vi "UHR-Fleezers Control (host) - 12.2.vi"() -> ()   [LabVIEW 2012] (continued)
      tunnel: [w2214] -> w1523 mode=indexing
      tunnel: w1485 -> [w2213]
      workers-P: _ -> [_]
      n1078 = Bundle By Name("Y"=w2218, "dt"=w2217) -> (w2219:waveform(dbl))  [unwired: 1 out]
      n1079 = Set Waveform Attribute(5:w2216, 6:w2215, 7:w2219) -> (3:w2214:waveform(dbl))  [unwired: 1 in, 2 out]
      n1080 = call "downsample 1D array - double.vi"("Ave N"=w2220, "Array In"=w2218) -> ("Array Out"=w2221:dbl[])  [unwired: 1 out]
      n1081 = Bundle By Name(cluster=w2214, "t0"=w2212, "Y"=w2221, "dt"=w2213) -> (w2222:waveform(dbl))
    }
    n1082 = Bundle("BD 1 Frequency 1 (MHz)"=w1439, "BD 1 Frequency 2 (MHz)"=w1438) -> (w1440:T41)  [unwired: 1 out]
    n1083 = call-poly <vilib>:"Mean.vi"("X"=w1473) -> ("mean"=w1461:dbl)  [unwired: 1 out]
    n1084 = call-poly <vilib>:"Mean.vi"("X"=w1474) -> ("mean"=w1462:dbl)  [unwired: 1 out]
    n1085 = Reciprocal(x=w1485) -> (1/x=→"Trap Disp. Freq. (Hz)":dbl)
    n1086 = Cluster To Array(cluster=w1440) -> (array=w1437:dbl[])
    n1087 = local read "Trap X AI1 (DMA)"() -> (w1472:T13)
    n1088 = local read "Data points/scans (MCL)"() -> (w1637:dbl)
    n1089 = To Fixed-Point(number=w1461) -> (fixed-point=w1459:fxp<+/-,16,1>)  [unwired: 1 in]
    n1090 = To Fixed-Point(number=w1462) -> (fixed-point=w1460:fxp<+/-,16,1>)  [unwired: 1 in]
    n1091 = Bundle("Trap 1 Pos.", "Trap 2 Pos.") -> (w1481:cluster{string, string})  [unwired: 1 out]
    n1092 = Bundle By Name(cluster=w1472, "Set 1"=w1460, "Set 2"=w1459) -> (→"Trap X AI1 (DMA)":T13)
    n1093 = Cluster To Array(cluster=w1481) -> (array=w1478:string[])
    n1094 = Bundle("APD 1", "APD 2") -> (w1658:cluster{string, string})  [unwired: 1 out]
    n1095 = Select(t=-1.0, s="Negate Y Axis", f=1.0) -> (s? t:f=w1422:dbl)
    n1096 = for "Trap Position" {
      tunnel: w1487 -> [w1854] mode=indexing
      tunnel: "Trap Pos. Disp. Downsample" -> [w1853]
      tunnel: w1403 -> [w1851]
      tunnel: w1483 -> [w1850]
      tunnel: w1482 -> [w1848]
      tunnel: w1478 -> [w1847] mode=indexing
      tunnel: [w1846] -> w1392 mode=indexing
      tunnel: w1437 -> [w1844] mode=indexing
      tunnel: w1436 -> [w1842]
      tunnel: w1422 -> [w1841]
      n1097 = call "downsample 1D array - double.vi"("Ave N"=w1853, "Array In"=w1854) -> ("Array Out"=w1852:dbl[])  [unwired: 1 out]
      n1098 = Subtract(x=w1852, y=w1844) -> (x-y=w1845:dbl[])
      n1099 = Multiply(x=w1842, y=w1845) -> (x*y=w1843:dbl[])
      n1100 = Multiply(x=w1841, y=w1843) -> (x*y=w1840:dbl[])
      n1101 = Bundle By Name("Y"=w1840, "dt"=w1851, "t0"=w1850) -> (w1849:waveform(dbl))  [unwired: 1 out]
      n1102 = Set Waveform Attribute(5:w1847, 6:w1848, 7:w1849) -> (3:w1846:waveform(dbl))  [unwired: 1 in, 2 out]
    }
    n1103 = Cluster To Array(cluster=w1658) -> (array=w1655:string[])
    n1104 = for "APD" {
      tunnel: w1626 -> [w2201] mode=indexing
      tunnel: w1512 -> [w2209]
      tunnel: [w2205] -> w1519 mode=indexing
      tunnel: "APD Disp. Scale" -> [w2206]
      tunnel: w1482 -> [w2204]
      tunnel: w1655 -> [w2203] mode=indexing
      tunnel: "APD Disp. Downsample" -> [w2199]
      tunnel: [w2202] -> w1654
      workers-P: _ -> [_]
      tunnel: w1483 -> [w2198]
      n1105 = call "integrate 1D array interval - double.vi"("Ave N"=w2199, "Array In"=w2201) -> ("Array Out"=w2200:dbl[])  [unwired: 1 out]
      n1106 = Multiply(x=w2209, y=w2199) -> (x*y=w2202:dbl)
      n1107 = Divide(x=w2200, y=w2206) -> (x/y=w2207:dbl[])
      n1108 = Bundle By Name("t0"=w2198, "Y"=w2207, "dt"=w2202) -> (w2208:waveform(dbl))  [unwired: 1 out]
      n1109 = Set Waveform Attribute(5:w2203, 6:w2204, 7:w2208) -> (3:w2205:waveform(dbl))  [unwired: 1 in, 2 out]
    }
    "APD Display Period (s)" <- w1654
    n1110 = Reciprocal(x=w1654) -> (1/x=→"APD Display Freq. (Hz)":dbl)
    n1111 = local read "Display Period (s)"() -> (w1543:dbl)
    n1112 = Increment(x=w1637) -> (x+1=w1638:dbl)
    n1113 = To Double Precision Float(number=w1555) -> (double precision float=w1554:dbl[])
    n1114 = Index Array(array=w1392, index=0) -> (element=w1396:waveform(dbl))
    n1115 = Index Array(array=w1392, index=1) -> (element=w1391:waveform(dbl))
    n1116 = feedback #7(w1638) -> (w1641:dbl)
    n1117 = Select(t=0, s=w1628, f=w1641) -> (s? t:f=w1634:dbl)
    n1118 = Array Size(array=w1554) -> (size(s)=w1640:i32)
    n1119 = Add(x=w1640, y=w1634) -> (x+y=w1635:dbl)
    n1120 = Unbundle By Name(w1396) -> ("Y"=w1397:dbl[])
    n1121 = feedback #8(w1555) -> (w1624:u32[])
    n1122 = Build Array (concatenate)(w1624, w1555) -> (w1621:u32[])
    n1123 = feedback #9(w1499) -> (w1518:u32[])
    n1124 = Divide(x="Bead Sep. Int. Time (s)", y=w1543) -> (x/y=w1432:dbl)
    n1125 = Build Array (concatenate)(w1518, w1499) -> (w1517:u32[])
    n1126 = Add(x=w1397, y="FB Trap Pos Offset") -> (x+y=w1395:dbl[])
    "T1 x pos data" <- w1395
    n1127 = Greater?(x=w1635, y=w1637) -> (0:w1636:bool)
    n1128 = feedback #10(w1395) -> (w1434:dbl[])
    n1129 = Build Array (concatenate)(w1395, w1434) -> (w1433:dbl[])
    n1130 = Bundle By Name(cluster=w1396, "Y"=w1395) -> (w1394:waveform(dbl))
    n1131 = Select(t=w1634, s=w1636, f=w1635) -> (s? t:f=w1633:dbl)
    n1132 = feedback-in #7(w1633) -> ()
    n1133 = Array Size(array=w1621) -> (size(s)=w1618:i32)
    n1134 = Array Size(array=w1555) -> (size(s)=w1620:i32)
    n1135 = local read "MCL Scanning"() -> (w1631:bool)
    n1136 = local read "APD Integration Time (s)"() -> (w1526:dbl)
    n1137 = Bundle(w1394, w1391) -> (w1390:cluster{waveform(dbl), waveform(dbl)})  [unwired: 1 out]
    n1138 = Build Array (concatenate)(w1519, w1659) -> (w1521:waveform(dbl)[])
    "All Signals" <- w1521
    n1139 = Split 1D Array(array=w1433, index=w1432) -> (first subarray=w1426:dbl[])  [unwired: 1 out]
    n1140 = feedback-in #10(w1426) -> ()
    n1141 = Multiply(x=w1620, y="APD Ave N") -> (x*y=w1619:dbl)
    n1142 = Greater?(x=w1618, y=w1619) -> (0:w1622:bool)
    n1143 = Not(x=w1636) -> (.not. x?=w1630:bool)
    n1144 = Cluster To Array(cluster=w1390) -> (array=w1366:waveform(dbl)[])
    "Trap Positions" <- w1366
    n1145 = To Double Precision Float(number=w1499) -> (double precision float=w1498:dbl[])
    n1146 = call-poly <vilib>:"Mean.vi"("X"=w1426) -> ("mean"=w1425:dbl)  [unwired: 1 out]
    "Mean T1 Position (nm)" <- w1425
    n1147 = Subtract(x=w1426, y=w1425) -> (x-y=w1431:dbl[])
    n1148 = Square(x=w1431) -> (x^2=w1430:dbl[])
    n1149 = And(x=w1630, y=w1631) -> (x .and. y?=w1632:bool)
    n1150 = call-poly <vilib>:"Mean.vi"("X"=w1430) -> ("mean"=w1429:dbl)  [unwired: 1 out]
    n1151 = case shown="True" w1622 {
      tunnel: w1621 -> [w1981 w1988]
      tunnel: [w1981 w1986] -> w1572
      tunnel: w1619 -> [_ w1983]
      tunnel: w1618 -> [_ w1987]
      tunnel: w1517 -> [w1980 w1985]
      tunnel: [w1980 w1982] -> w1514
      frame False {
      }
      frame True {
        n1152 = Subtract(x=w1987, y=w1983) -> (x-y=w1984:dbl)
        n1153 = Array Subset(array=w1988, index=w1984, length=w1983) -> (w1986:u32[])
        n1154 = Array Subset(array=w1985, index=w1984, length=w1983) -> (w1982:u32[])
      }
    }
    n1155 = feedback-in #8(w1572) -> ()
    n1156 = feedback-in #9(w1514) -> ()
    n1157 = Square Root(x=w1429) -> (sqrt(x)=w1428:dbl)
    n1158 = Or(x=w1632, y=w1628) -> (x .or. y?=w1629:bool)
    n1159 = Equal?(x="Tab Control 6", y=T29."High Res Display") -> (x = y?=w1561:bool)
    n1160 = Multiply(x="APD Disp. Scale", y=w1519) -> (x*y=w1528:waveform(dbl)[])
    n1161 = Multiply(x=10.0, y=w1428) -> (x*y=→"Trap 1 Position RMS (A)":dbl)
    n1162 = Multiply(x="APD Disp. Downsample", y=w1526) -> (x*y=w1524:dbl)
    n1163 = Divide(x=w1528, y=w1524) -> (x/y=w1496:waveform(dbl)[])
    n1164 = case "For displaying the high resolution display (no downsampling)" shown="True" w1561 {
      tunnel: w1523 -> [_ w1874]
      frame False {
      }
      frame True {
        n1165 = Index Array(array=w1874, index="High Res. Display") -> (element=w1875:waveform(dbl))
        n1166 = call <vilib>:"Std Deviation and Variance.vi"("X"=w1875) -> ("mean"=w1882:dbl, "standard deviation"=w1887:dbl)  [unwired: 1 in, 1 out]
        "Mean Intensity" <- w1882
        "Sigma" <- w1887
        n1167 = Subtract(x=w1875, y=w1882) -> (x-y=w1881:waveform(dbl))
        n1168 = Select(t=w1881, s="Subtract mean", f=w1875) -> (s? t:f=→"1 Channel":waveform(dbl))
        n1169 = Divide(x=w1887, y=w1882) -> (x/y=→"Sigma/Mean":dbl)
        n1170 = feedback #11(1) -> (w1876:i32)
        n1171 = Greater Or Equal?(x=w1876, y="Slow mean N ave.") -> (x >= y?=w1889:bool)
        n1172 = Increment(x=w1876) -> (x+1=w1891:i32)
        n1173 = Select(t=1, s=w1889, f=w1891) -> (s? t:f=w1878:i32)
        n1174 = feedback-in #11(w1878) -> ()
        n1175 = feedback #12() -> (w1879:waveform(dbl))  [unwired: 1 out]
        n1176 = case shown="Default" w1876 {
          tunnel: [w1894 w1897] -> w1880
          tunnel: w1879 -> [w1896 _]
          tunnel: w1875 -> [w1895 w1897]
          frame Default {
            n1177 = call-poly <vilib>:"Append Waveforms.vi"("waveform B"=w1895, "waveform A"=w1896) -> ("waveform out"=w1894:waveform(dbl))  [unwired: 1 in, 8 out]
          }
          frame 1 {
          }
        }
        n1178 = feedback-in #12(w1880) -> ()
        n1179 = case shown="True" w1889 {
          tunnel: w1880 -> [_ w1893]
          frame False {
          }
          frame True {
            n1180 = call-poly <vilib>:"Mean.vi"("X"=w1893) -> ("mean"=→"Slow mean":dbl)  [unwired: 1 out]
          }
        }
      }
    }
    n1181 = Index Array(array=w1496, index=0) -> (element=w1506:waveform(dbl))
    n1182 = Index Array(array=w1496, index=1) -> (element=w1504:waveform(dbl))
    n1183 = case "For computing FFTs for display" shown="True" "Compute FFT" {
      tunnel: w1523 -> [_ w2600]
      frame False {
      }
      frame True {
        n1184 = Build Array("FFT 1 Choice 1", "FFT 1 Choice 2", "FFT 2 Choice 1", "FFT 2 Choice 2") -> (w2593:u16[])
        n1185 = Array Size(array=w2600) -> (size(s)=w2599:i32)
        n1186 = feedback-in #13(w2593) -> ()
        n1187 = feedback #13(u16[] [100, 100, 100, 100]) -> (w2594:u16[])
        n1188 = feedback-in #14("# Spectra to Ave.") -> ()
        n1189 = feedback #14("# Spectra to Ave.") -> (w2591:dbl)
        n1190 = Not Equal?(x="# Spectra to Ave.", y=w2591) -> (x != y?=w2590:bool)
        n1191 = Not Equal?(x=w2593, y=w2594) -> (x != y?=w2592:bool)
        n1192 = feedback #15(1.0) -> (w2577:dbl)
        n1193 = Compound Arithmetic op=OR("Reset FFT", w2592, w2590) -> (w2575:bool)
        n1194 = Select(t=1.0, s=w2575, f=w2577) -> (s? t:f=w2579:dbl)
        n1195 = Greater?(x=w2579, y="# Spectra to Ave.") -> (0:w2598:bool)
        n1196 = Increment(x=w2579) -> (x+1=w2578:dbl)
        n1197 = feedback-in #15(w2578) -> ()
        n1198 = local read "DMA Update Period (s)"() -> (w2573:dbl)
        n1199 = Multiply(x="# Spectra to Ave.", y=w2573) -> (x*y=→"Ave. Time (s)":dbl)
        n1200 = Build Array(cluster{"f0":dbl, "df":dbl, "magnitude":dbl[]} {"f0"=0.0, "df"=0.0, "magnitude"=[]} ("PSD")) -> (w2582:cluster{"f0":dbl, "df":dbl, "magnitude":dbl[]}[])
        n1201 = Build Array(w2582, w2582, w2582, w2582) -> (w2584:T42)
        n1202 = feedback #16(w2584) -> (w2589:T42)
        n1203 = for {
          N: 4 -> [_]
          tunnel: w2593 -> [w2622] mode=indexing
          tunnel: w2600 -> [w2623]
          tunnel: w2599 -> [w2625]
          tunnel: w2575 -> [w2618]
          tunnel: w2598 -> [w2617]
          tunnel: "# Spectra to Ave." -> [w2616]
          tunnel: [w2615] -> w2588 mode=indexing
          tunnel: w2589 -> [w2620] mode=indexing
          tunnel: [w2619] -> w2576 mode=indexing
          tunnel: w2579 -> [w2614]
          n1204 = Less?(x=w2622, y=w2625) -> (x < y?=w2624:bool)
          n1205 = Index Array(array=w2623, index=w2622) -> (element=w2621:waveform(dbl))
          n1206 = case shown="True" w2624 {
            tunnel: w2621 -> [_ w2642]
            tunnel: w2620 -> [w2627 w2640]
            tunnel: [w2627 w2628] -> w2619
            tunnel: w2618 -> [_ w2639]
            tunnel: w2617 -> [_ w2632]
            tunnel: w2616 -> [_ w2631]
            tunnel: [cluster{"f0":dbl, "df":dbl, "magnitude":dbl[]} {"f0"=0.0, "df"=0.0, "magnitude"=[]} ("PSD") w2633] -> w2615
            tunnel: w2614 -> [_ w2630]
            frame False {
            }
            frame True {
              n1207 = call <vilib>:"Std Deviation and Variance.vi"("X"=w2642) -> ("mean"=w2643:dbl)  [unwired: 1 in, 2 out]
              n1208 = Subtract(x=w2642, y=w2643) -> (x-y=w2641:waveform(dbl))
              n1209 = xnode "Spectral Measurements"("Signals"=w2641) -> ("PSD"=w2635:cluster{"f0":dbl, "df":dbl, "magnitude":dbl[]})  [unwired: 1 in, 1 out]
              n1210 = case shown="False" w2639 {
                tunnel: w2640 -> [w2652 _]
                tunnel: [w2648 w2657] -> w2628
                tunnel: w2635 -> [w2651 w2658]
                tunnel: w2632 -> [w2650 _]
                frame False {
                  n1211 = Build Array (concatenate)(w2652, w2651) -> (w2649:cluster{"f0":dbl, "df":dbl, "magnitude":dbl[]}[])
                  n1212 = case shown="True" w2650 {
                    tunnel: w2649 -> [w2653 w2656]
                    tunnel: [w2653 w2654] -> w2648
                    frame False {
                    }
                    frame True {
                      n1213 = Delete From Array(array=w2656, index=0) -> (array with subset deleted=w2654:cluster{"f0":dbl, "df":dbl, "magnitude":dbl[]}[])  [unwired: 1 in, 1 out]
                    }
                  }
                }
                frame True {
                  n1214 = Build Array(w2658) -> (w2657:cluster{"f0":dbl, "df":dbl, "magnitude":dbl[]}[])
                }
              }
              n1215 = for {
                tunnel: w2628 -> [w2647] mode=indexing
                tunnel: [w2646] -> w2638 mode=indexing
                workers-P: _ -> [_]
                n1216 = Unbundle By Name(w2647) -> ("magnitude"=w2646:dbl[])
              }
              n1217 = Transpose 2D Array(2D array=w2638) -> (transposed array=w2637:dbl[][])
              n1218 = for {
                tunnel: w2637 -> [w2645] mode=indexing
                tunnel: [w2644] -> w2636 mode=indexing
                workers-P: _ -> [_]
                n1219 = Add Array Elements(numeric array=w2645) -> (sum=w2644:dbl)
              }
              n1220 = Select(t=w2631, s=w2632, f=w2630) -> (s? t:f=w2629:dbl)
              n1221 = Divide(x=w2636, y=w2629) -> (x/y=w2634:dbl[])
              n1222 = Bundle By Name(cluster=w2635, "magnitude"=w2634) -> (w2633:cluster{"f0":dbl, "df":dbl, "magnitude":dbl[]})
            }
          }
        }
        n1223 = case shown="True" w2575 {
          tunnel: w2576 -> [w2607 w2613]
          tunnel: [w2607 w2608] -> w2574
          frame False {
          }
          frame True {
            n1224 = Array Subset(array=w2613, index (row)=0 ("index"), length (row)=4 ("length"), index (col)=0 ("index"), length (col)=1 ("length")) -> (w2608:T42)
          }
        }
        n1225 = feedback-in #16(w2574) -> ()
        n1226 = Split 1D Array(array=w2588, index=2) -> (first subarray=→"FFT 1":cluster{"f0":dbl, "df":dbl, "magnitude":dbl[]}[], second subarray=→"FFT 2":cluster{"f0":dbl, "df":dbl, "magnitude":dbl[]}[])
      }
    }
    n1227 = case "For plotting results of scanning MCL" shown="True" w1629 {
      tunnel: w1628 -> [_ w2021]
      tunnel: w1554 -> [_ w2117]
      tunnel: w1637 -> [_ _]
      tunnel: w1523 -> [_ w2091]
      tunnel: w1498 -> [_ w2022]
      tunnel: w1497 -> [_ w1995]
      frame False {
      }
      frame True {
        w2002 = u32 0 items=["Horizontal", "Vertical", "Central", "1st Diagonal", "2nd Diagonal"] ("Type of Symmetry")
        w2030 = u32 0 items=["Horizontal", "Vertical", "Central", "1st Diagonal", "2nd Diagonal"] ("Type of Symmetry")
        w2033 = u32 0 items=["Horizontal", "Vertical", "Central", "1st Diagonal", "2nd Diagonal"] ("Type of Symmetry")
        w2062 = u32 0 items=["Horizontal", "Vertical", "Central", "1st Diagonal", "2nd Diagonal"] ("Type of Symmetry")
        n1228 = Index Array(array=w2091, index=10) -> (element=w2097:waveform(dbl))
        n1229 = Index Array(array=w2091, index=11) -> (element=w2094:waveform(dbl))
        n1230 = local read "Cycles/step (MCL)"() -> (w2047:u64)
        n1231 = Index Array(array=w2091, index="Channel") -> (element=w2093:waveform(dbl))
        n1232 = Unbundle(w1995) -> ("New Image"=w1994:T2, "New Image"=w1993:T2, "New Image"=w1992:T2, "New Image"=w1991:T2)
        n1233 = Unbundle By Name(w2097) -> ("Y"=w2049:dbl[])
        n1234 = Unbundle By Name(w2094) -> ("Y"=w2051:dbl[])
        n1235 = Unbundle By Name(w2093) -> ("Y"=w2056:dbl[])
        n1236 = call "downsample 1D array - double.vi"("Ave N"=w2047, "Array In"=w2049) -> ("Array Out"=w2048:dbl[])  [unwired: 1 out]
        n1237 = call "downsample 1D array - double.vi"("Ave N"=w2047, "Array In"=w2051) -> ("Array Out"=w2050:dbl[])  [unwired: 1 out]
        n1238 = call "downsample 1D array - double.vi"("Ave N"=w2047, "Array In"=w2056) -> ("Array Out"=w2055:dbl[])  [unwired: 1 out]
        n1239 = feedback #17(w2117) -> (w2118:dbl[])
        n1240 = Build Array (concatenate)(w2118, w2117) -> (w2099:dbl[])
        n1241 = feedback #18(w2022) -> (w2024:dbl[])
        n1242 = Build Array (concatenate)(w2024, w2022) -> (w2023:dbl[])
        n1243 = local read "Scan steps (MCL)"() -> (w2004:u64)
        n1244 = Select(t=w2117, s=w2021, f=w2099) -> (s? t:f=w2103:dbl[])
        n1245 = feedback-in #17(w2103) -> ()
        n1246 = Select(t=w2022, s=w2021, f=w2023) -> (s? t:f=w2005:dbl[])
        n1247 = feedback-in #18(w2005) -> ()
        n1248 = local read "Scan lines (y)"() -> (w1990:u64)
        n1249 = local read "N APD Samp/step"() -> (w2006:dbl)
        n1250 = feedback #19(w2048) -> (w2105:dbl[])
        n1251 = Build Array (concatenate)(w2105, w2048) -> (w2096:dbl[])
        n1252 = feedback #20(w2055) -> (w2115:dbl[])
        n1253 = Build Array (concatenate)(w2115, w2055) -> (w2114:dbl[])
        n1254 = feedback #21(w2050) -> (w2107:dbl[])
        n1255 = Build Array (concatenate)(w2107, w2050) -> (w2108:dbl[])
        n1256 = Select(t=w2048, s=w2021, f=w2096) -> (s? t:f=w2052:dbl[])
        n1257 = feedback-in #19(w2052) -> ()
        n1258 = Select(t=w2055, s=w2021, f=w2114) -> (s? t:f=w2054:dbl[])
        n1259 = feedback-in #20(w2054) -> ()
        n1260 = Select(t=w2050, s=w2021, f=w2108) -> (s? t:f=w2053:dbl[])
        n1261 = feedback-in #21(w2053) -> ()
        n1262 = Multiply(x=w2004, y=u64 2) -> (x*y=w1989:u64)
        n1263 = call "integrate 1D array interval - double.vi"("Ave N"=w2006, "Array In"=w2005) -> ("Array Out"=w2017:dbl[])  [unwired: 1 out]
        n1264 = call "integrate 1D array interval - double.vi"("Ave N"=w2006, "Array In"=w2103) -> ("Array Out"=w2102:dbl[])  [unwired: 1 out]
        n1265 = Array Size(array=w2017) -> (size(s)=w2018:i32)
        n1266 = Array Size(array=w2102) -> (size(s)=w2104:i32)
        n1267 = Multiply(x=w1990, y=w1989) -> (x*y=w2020:u64)
        n1268 = Multiply(x=w1990, y=w1989) -> (x*y=w2112:u64)
        n1269 = call-poly <vilib>:"Mean.vi"("X"=w2052) -> ("mean"=w2036:dbl)  [unwired: 1 out]
        n1270 = Subtract(x=w2020, y=w2018) -> (x-y=w2011:u64)
        n1271 = call-poly <vilib>:"Mean.vi"("X"=w2054) -> ("mean"=w2041:dbl)  [unwired: 1 out]
        n1272 = call-poly <vilib>:"Mean.vi"("X"=w2053) -> ("mean"=w2039:dbl)  [unwired: 1 out]
        n1273 = call-poly <vilib>:"Mean.vi"("X"=w2017) -> ("mean"=w2008:dbl)  [unwired: 1 out]
        n1274 = Subtract(x=w2112, y=w2104) -> (x-y=w2046:u64)
        n1275 = call-poly <vilib>:"Mean.vi"("X"=w2102) -> ("mean"=w2043:dbl)  [unwired: 1 out]
        n1276 = Initialize Array(1.0 ("element"), w2011) -> (w2007:dbl[])
        n1277 = Initialize Array(1.0 ("element"), w2046) -> (w2037:dbl[])
        n1278 = Multiply(x=w2007, y=w2008) -> (x*y=w2009:dbl[])
        n1279 = Multiply(x=w2037, y=w2039) -> (x*y=w2040:dbl[])
        n1280 = Multiply(x=w2037, y=w2041) -> (x*y=w2042:dbl[])
        n1281 = Multiply(x=w2037, y=w2036) -> (x*y=w2038:dbl[])
        n1282 = Multiply(x=w2037, y=w2043) -> (x*y=w2044:dbl[])
        n1283 = Build Array (concatenate)(w2052, w2038) -> (w2106:dbl[])
        n1284 = Build Array (concatenate)(w2054, w2042) -> (w2110:dbl[])
        n1285 = Build Array (concatenate)(w2053, w2040) -> (w2109:dbl[])
        n1286 = Build Array (concatenate)(w2017, w2009) -> (w2019:dbl[])
        n1287 = Build Array (concatenate)(w2102, w2044) -> (w2111:dbl[])
        n1288 = Reshape Array(w2106, w1990, w1989) -> (w2072:dbl[][])
        n1289 = Reshape Array(w2019, w1990, w1989) -> (w2015:dbl[][])
        n1290 = Reshape Array(w2110, w1990, w1989) -> (w2064:dbl[][])
        n1291 = Reshape Array(w2109, w1990, w1989) -> (w2079:dbl[][])
        n1292 = Reshape Array(w2111, w1990, w1989) -> (w2089:dbl[][])
        n1293 = Array Subset(array=w2079, index (col)=0 ("index"), length (col)=w2004) -> (w2084:dbl[][])  [unwired: 2 in]
        n1294 = Array Subset(array=w2079, index (col)=w2004) -> (w2082:dbl[][])  [unwired: 3 in]
        n1295 = Array Subset(array=w2064, index (col)=0 ("index"), length (col)=w2004) -> (w2070:dbl[][])  [unwired: 2 in]
        n1296 = Array Subset(array=w2064, index (col)=w2004) -> (w2068:dbl[][])  [unwired: 3 in]
        n1297 = Array Subset(array=w2015, index (col)=0 ("index"), length (col)=w2004) -> (w2014:dbl[][])  [unwired: 2 in]
        n1298 = Array Subset(array=w2015, index (col)=w2004) -> (w2012:dbl[][])  [unwired: 3 in]
        n1299 = Array Subset(array=w2089, index (col)=0 ("index"), length (col)=w2004) -> (w2088:dbl[][])  [unwired: 2 in]
        n1300 = Array Subset(array=w2089, index (col)=w2004) -> (w2086:dbl[][])  [unwired: 3 in]
        n1301 = Array Subset(array=w2072, index (col)=0 ("index"), length (col)=w2004) -> (w2077:dbl[][])  [unwired: 2 in]
        n1302 = Array Subset(array=w2072, index (col)=w2004) -> (w2075:dbl[][])  [unwired: 3 in]
        n1303 = for {
          tunnel: w2084 -> [w2126] mode=indexing
          tunnel: [w2125] -> w2083 mode=indexing
          workers-P: _ -> [_]
          n1304 = Reverse 1D Array(array=w2126) -> (reversed array=w2125:dbl[])
        }
        n1305 = for {
          tunnel: w2070 -> [w2122] mode=indexing
          tunnel: [w2121] -> w2069 mode=indexing
          workers-P: _ -> [_]
          n1306 = Reverse 1D Array(array=w2122) -> (reversed array=w2121:dbl[])
        }
        n1307 = for {
          tunnel: w2014 -> [w2120] mode=indexing
          tunnel: [w2119] -> w2013 mode=indexing
          workers-P: _ -> [_]
          n1308 = Reverse 1D Array(array=w2120) -> (reversed array=w2119:dbl[])
        }
        n1309 = for {
          tunnel: w2088 -> [w2128] mode=indexing
          tunnel: [w2127] -> w2087 mode=indexing
          workers-P: _ -> [_]
          n1310 = Reverse 1D Array(array=w2128) -> (reversed array=w2127:dbl[])
        }
        n1311 = for {
          tunnel: w2077 -> [w2124] mode=indexing
          tunnel: [w2123] -> w2076 mode=indexing
          workers-P: _ -> [_]
          n1312 = Reverse 1D Array(array=w2124) -> (reversed array=w2123:dbl[])
        }
        n1313 = Index Array(array=w2089, index (row)=0) -> (element=→"Waveform Graph":dbl[])  [unwired: 1 in]
        n1314 = Add(x=w2083, y=w2082) -> (x+y=w2081:dbl[][])
        n1315 = Add(x=w2069, y=w2068) -> (x+y=w2067:dbl[][])
        n1316 = Add(x=w2013, y=w2012) -> (x+y=w1997:dbl[][])
        n1317 = Add(x=w2087, y=w2086) -> (x+y=w2061:dbl[][])
        n1318 = Add(x=w2076, y=w2075) -> (x+y=w2074:dbl[][])
        n1319 = Divide(x=w2067, y=2) -> (x/y=w2065:dbl[][])
        n1320 = Divide(x=w2081, y=2) -> (x/y=w2026:dbl[][])
        n1321 = Divide(x=w2074, y=2) -> (x/y=w2028:dbl[][])
        n1322 = To Single Precision Float(number=w2061) -> (single precision float=w2060:sgl[][])
        n1323 = Transpose 2D Array(2D array=w2065) -> (transposed array=→"Data map":dbl[][])
        n1324 = To Single Precision Float(number=w1997) -> (single precision float=w2001:sgl[][])
        n1325 = To Single Precision Float(number=w2026) -> (single precision float=w2032:sgl[][])
        n1326 = To Single Precision Float(number=w2028) -> (single precision float=w2029:sgl[][])
        n1327 = call "IMAQ ArrayToImage"("Image Pixels (Float)"=w2060, "Image"=w1994) -> ("Image Out"=w2063:T2)  [unwired: 8 in, 1 out]
        n1328 = call "IMAQ ArrayToImage"("Image Pixels (Float)"=w2001, "Image"=w1993) -> ("Image Out"=w2003:T2)  [unwired: 8 in, 1 out]
        n1329 = call "IMAQ ArrayToImage"("Image Pixels (Float)"=w2032, "Image"=w1992) -> ("Image Out"=w2034:T2)  [unwired: 8 in, 1 out]
        n1330 = call "IMAQ ArrayToImage"("Image Pixels (Float)"=w2029, "Image"=w1991) -> ("Image Out"=w2031:T2)  [unwired: 8 in, 1 out]
        n1331 = call "IMAQ Symmetry"("Type of Symmetry"=w2062, "Image Src"=w2063) -> ("Image Dst Out"=w2058:T2)  [unwired: 3 in, 1 out]
        n1332 = call "IMAQ Symmetry"("Type of Symmetry"=w2002, "Image Src"=w2003) -> ("Image Dst Out"=w1999:T2)  [unwired: 3 in, 1 out]
        n1333 = call "IMAQ Symmetry"("Type of Symmetry"=w2033, "Image Src"=w2034) -> ("Image Dst Out"=→"Detection Laser X":T2)  [unwired: 3 in, 1 out]
        n1334 = call "IMAQ Symmetry"("Type of Symmetry"=w2030, "Image Src"=w2031) -> ("Image Dst Out"=→"Detection Laser Y":T2)  [unwired: 3 in, 1 out]
        n1335 = call "IMAQ Set Simple Calibration"("Calibration Axis Info"=T30 {"Origin Pixel"={"X"=0.0, "Y"=0.0}, "Angle Relative to Horizontal (deg)"=0.0, "Axis Reference"=0}, "Grid Descriptor"=T31 {"X Step"=0.3, "Y Step"=0.3, "Unit"=enum."Undefined"}, "Image"=w2058) -> ("Calibrated Image"=→"APD 1":T2)  [unwired: 7 in, 1 out]
        n1336 = call "IMAQ Set Simple Calibration"("Calibration Axis Info"=T30 {"Origin Pixel"={"X"=0.0, "Y"=0.0}, "Angle Relative to Horizontal (deg)"=0.0, "Axis Reference"=0}, "Grid Descriptor"=T31 {"X Step"=0.3, "Y Step"=0.3, "Unit"=enum."Undefined"}, "Image"=w1999) -> ("Calibrated Image"=→"APD 2":T2)  [unwired: 7 in, 1 out]
      }
    }
    n1337 = Subtract(x=w1504, y="APD 2 Offset") -> (x-y=w1501:waveform(dbl))
    n1338 = Subtract(x=w1506, y="APD 1 Offset") -> (x-y=w1502:waveform(dbl))
    n1339 = Index Array(array=w1521, index=3) -> (element=w1581:waveform(dbl))
    n1340 = Index Array(array=w1521, index=6) -> (element=w1578:waveform(dbl))
    n1341 = Build Array(w1502, w1501) -> (→"APD Chart":waveform(dbl)[])
    n1342 = Array Size(array=w1572) -> (size(s)=w1617:i32)
    n1343 = call <vilib>:"Std Deviation and Variance.vi"("X"=w1514) -> ("standard deviation"=w1513:dbl)  [unwired: 1 in, 2 out]
    n1344 = Add Array Elements(numeric array=w1514) -> (sum=w1516:u32)
    n1345 = Add Array Elements(numeric array=w1572) -> (sum=w1627:u32)
    n1346 = call <vilib>:"Std Deviation and Variance.vi"("X"=w1572) -> ("standard deviation"=w1571:dbl)  [unwired: 1 in, 2 out]
    n1347 = Divide(x="T1 offset_x (mV)", y=1000.0) -> (x/y=w1582:dbl)
    n1348 = Divide(x=w1513, y=w1512) -> (x/y=w1509:dbl)
    "Rate sigma (Hz) 2" <- w1509
    n1349 = Multiply(x=w1512, y=w1617) -> (x*y=w1515:dbl)
    "Int. Time (s)" <- w1515
    n1350 = Divide(x=w1516, y=w1515) -> (x/y=w1510:dbl)
    "APD 2 Rate (Hz)" <- w1510
    n1351 = Divide(x=w1627, y=w1515) -> (x/y=w1569:dbl)
    "APD 1 Rate (Hz)" <- w1569
    n1352 = Divide(x=w1571, y=w1512) -> (x/y=w1570:dbl)
    "Rate sigma (Hz)" <- w1570
    n1353 = Divide(x=w1509, y=w1510) -> (x/y=→"Sigma/Mean 2":dbl)
    n1354 = Divide(x=w1570, y=w1569) -> (x/y=→"Sigma/Mean":dbl)
    n1355 = feedback-in #22("Calibration") -> ()
    n1356 = feedback #22(u16 1 ("Calibration")) -> (w1600:u16)
    n1357 = Divide(x="T2 offset_x (mV)", y=1000.0) -> (x/y=w1580:dbl)
    n1358 = case shown="0, Default" "Calibration" {
      tunnel: "T1 alpha_x (nm/V)" -> [_ w1957 w1978]
      tunnel: "T1 kappa_x (pN/nm)" -> [_ _ w1968]
      tunnel: "T2 alpha_x (nm/V)" -> [_ w1956 w1976]
      tunnel: "T2 kappa_x (pN/nm)" -> [_ _ w1969]
      tunnel: w1581 -> [w1939 w1954 w1974]
      tunnel: w1578 -> [w1938 w1952 w1972]
      tunnel: [w1939 w1951 w1971] -> w1609
      tunnel: [w1938 w1950 w1970] -> w1608
      tunnel: ["T1 X (V)" ("Label.Text") "T1 X (nm)" ("Label.Text") "T1 X (pN)" ("Label.Text")] -> w1597
      tunnel: ["T2 X (V)" ("Label.Text") "T2 X (nm)" ("Label.Text") "T2 X (pN)" ("Label.Text")] -> w1596
      tunnel: ["Position (V)" ("Label.Text") "Position (nm)" ("Label.Text") "Force (pN)" ("Label.Text")] -> w1598
      tunnel: w1580 -> [_ w1942 w1961]
      tunnel: w1582 -> [_ w1945 w1963]
      tunnel: ["Mean (V)" ("Label.Text") "Mean (nm)" ("Label.Text") "Mean (pN)" ("Label.Text")] -> w1593
      tunnel: ["Difference (V)" ("Label.Text") "Difference (nm)" ("Label.Text") "Difference (pN)" ("Label.Text")] -> w1529
      frame 0, Default {
      }
      frame 1 {
        n1359 = Unbundle By Name(w1954) -> ("Y"=w1958:dbl[])
        n1360 = Unbundle By Name(w1952) -> ("Y"=w1943:dbl[])
        n1361 = Subtract(x=w1958, y=w1945) -> (x-y=w1946:dbl[])
        n1362 = Subtract(x=w1943, y=w1942) -> (x-y=w1944:dbl[])
        n1363 = Multiply(x=w1944, y=w1956) -> (x*y=w1953:dbl[])
        n1364 = Multiply(x=w1957, y=w1946) -> (x*y=w1955:dbl[])
        n1365 = Bundle By Name(cluster=w1952, "Y"=w1953) -> (w1950:waveform(dbl))
        n1366 = Bundle By Name(cluster=w1954, "Y"=w1955) -> (w1951:waveform(dbl))
      }
      frame 2 {
        n1367 = Unbundle By Name(w1974) -> ("Y"=w1979:dbl[])
        n1368 = Unbundle By Name(w1972) -> ("Y"=w1977:dbl[])
        n1369 = Subtract(x=w1977, y=w1961) -> (x-y=w1962:dbl[])
        n1370 = Subtract(x=w1979, y=w1963) -> (x-y=w1964:dbl[])
        n1371 = Compound Arithmetic op=MULTIPLY(w1962, w1976, w1969) -> (w1973:dbl[])
        n1372 = Compound Arithmetic op=MULTIPLY(w1968, w1978, w1964) -> (w1975:dbl[])
        n1373 = Bundle By Name(cluster=w1972, "Y"=w1973) -> (w1970:waveform(dbl))
        n1374 = Bundle By Name(cluster=w1974, "Y"=w1975) -> (w1971:waveform(dbl))
      }
    }
    n1375 = Not Equal?(x=w1600, y="Calibration") -> (x != y?=w1559:bool)
    n1376 = case shown="True" w1559 {
      tunnel: w1598 -> [_ w1932]
      tunnel: w1597 -> [_ w1931]
      tunnel: w1596 -> [_ w1930]
      tunnel: w1593 -> [_ w1929]
      tunnel: w1529 -> [_ w1928]
      frame False {
      }
      frame True {
        n1377 = property on="Force" class="WFChart (strict)"("YScale.NameLbl.Text"=w1932) -> ()  [unwired: 2 in, 2 out]
        n1378 = property on="T2 X" class="DigNum (strict)"("Caption.Text"=w1930) -> ()  [unwired: 2 in, 2 out]
        n1379 = property on="T1 X" class="DigNum (strict)"("Caption.Text"=w1931) -> ()  [unwired: 2 in, 2 out]
        n1380 = property on="Mean" class="DigNum (strict)"("Caption.Text"=w1929) -> ()  [unwired: 2 in, 2 out]
        n1381 = property on="Difference" class="DigNum (strict)"("Caption.Text"=w1928) -> ()  [unwired: 2 in, 2 out]
      }
    }
    n1382 = Unbundle By Name(w1581) -> ("Y"=w1584:dbl[])
    n1383 = Unbundle By Name(w1578) -> ("Y"=w1587:dbl[])
    n1384 = Subtract(x=w1584, y=w1582) -> (x-y=w1585:dbl[])
    n1385 = Subtract(x=w1587, y=w1580) -> (x-y=w1586:dbl[])
    n1386 = Multiply(x=w1586, y="T2 alpha_x (nm/V)") -> (x*y=w1371:dbl[])
    n1387 = Multiply(x="T1 alpha_x (nm/V)", y=w1585) -> (x*y=w1372:dbl[])
    n1388 = Not(x="Trap Trig. Fl.") -> (.not. x?=w1408:bool)
    n1389 = Multiply(x=w1608, y=-1.0) -> (x*y=w1589:waveform(dbl))
    n1390 = Subtract(x=w1372, y=w1371) -> (x-y=w1577:dbl[])
    n1391 = Unbundle By Name(w1608) -> ("Y"=w1548:dbl[])
    n1392 = Unbundle By Name(w1609) -> ("Y"=w1373:dbl[])
    n1393 = Negate(x=w1577) -> (-x=w1369:dbl[])
    n1394 = Build Array(w1609, w1589) -> (→"Force":waveform(dbl)[])
    n1395 = Subtract(x=w1369, y="Offset (nm)") -> (x-y=w1546:dbl[])
    n1396 = case shown="True" "Read Lateness and Rel Phase" {
      tunnel: w1389 -> [w1898 w1927]
      tunnel: w1388 -> [w1899 w1926]
      tunnel: [w1898 w1925] -> w1575
      tunnel: [w1899 w1924] -> w1574
      frame False {
      }
      frame True {
        n1397 = xnode "Read/Write Control"("FPGA VI Reference In"=w1927, "error in"=w1926) -> ("FPGA VI Reference Out"=w1925:T19, "error out"=w1924:errorcluster, "GI Relative phase"=→"GI relative phase":i16, "Relative phase"=→"Relative phase (AI1)":i16, "AI Late Counter"=→"Late Counter (AI1)":u8, "GI Late Counter"=→"GI Late Counter":u8, "MCL Late Counter"=→"MCL Late Counter":u8, "MCL Relative Phase"=→"Relative Phase (MCL)":i16, "APD Acq Relative Phase"=→"APD Acq Relative Phase":i16, "APD 1 Gate Relative Phase"=→"APD 1 Gate Relative Phase":i16, "APD 2 Gate Relative Phase"=→"APD 2 Gate Relative Phase":i16, "APD Acq Late Counter"=→"APD Acq Late Counter":u8, "APD 1 Gate Late Counter"=→"APD 1 Gate Late Counter":u8, "APD 2 Gate Late Counter"=→"APD 2 Gate Late Counter":u8, "Green FB Relative Phase"=→"Relative phase (Green FB)":i16, "GI Relative phase 2"=→"GI relative phase 2":i16, "GI Late Counter 2"=→"GI Late Counter 2":u8, "Trap Pos FIFO Timeout"=→"Trap Pos FIFO Timeout":u16, "Trap AI FIFO Timeout"=→"Trap AI FIFO Timeout":u16, "RI Late Counter"=→"RI Late Counter":u8, "RI Late Counter 2"=→"RI Late Counter 2":u8, "RI Relative phase"=→"RI relative phase":i16, "RI Relative phase 2"=→"RI relative phase 2":i16, "Red FB Relative Phase"=→"Relative phase (RI FB)":i16, "Red Late Counter"=→"Red AI Late Counter":u8, "Green Late Counter"=→"Green AI Late Counter":u8)
      }
    }
    n1398 = call-poly <vilib>:"Mean.vi"("X"=w1548) -> ("mean"=w1375:dbl)  [unwired: 1 out]
    "T2 X" <- w1375
    n1399 = Negate(x=w1548) -> (-x=w1549:dbl[])
    n1400 = call-poly <vilib>:"Mean.vi"("X"=w1373) -> ("mean"=w1376:dbl)  [unwired: 1 out]
    "T1 X" <- w1376
    n1401 = Negate(x=w1375) -> (-x=w1374:dbl)
    n1402 = Bundle By Name(cluster=w1581, "Y"=w1546) -> (w1520:waveform(dbl))
    "Bead Separation" <- w1520
    n1403 = Add(x=w1373, y=w1549) -> (x+y=w1550:dbl[])
    n1404 = Add(x=w1376, y=w1374) -> (x+y=w1595:dbl)
    n1405 = Subtract(x=w1376, y=w1374) -> (x-y=→"Difference":dbl)
    n1406 = Divide(x=w1550, y=2.0) -> (x/y=→"Vec Mean of T1 T2":dbl[])
    n1407 = Divide(x=w1595, y=2.0) -> (x/y=w1552:dbl)
    "Mean" <- w1552
    n1408 = feedback-in #23("Trap Trig. Fl.") -> ()
    n1409 = feedback #23("Trap Trig. Fl.") -> (w1406:bool)
    n1410 = And(x=w1408, y=w1406) -> (x .and. y?=w1407:bool)
    n1411 = case "If have just turned off triggering" shown="True" w1407 {
      tunnel: w1389 -> [_ w1733]
      tunnel: w1388 -> [_ w1732]
      frame False {
      }
      frame True {
        w1731 = FALSE ("FPGA Trap Trig")
        n1412 = xnode "Read/Write Control"("FPGA VI Reference In"=w1733, "error in"=w1732, "FPGA Trap Trig"=w1731) -> ("FPGA VI Reference Out"=w1730:T19, "error out"=w1729:errorcluster)
        n1413 = xnode "Read/Write Control"("FPGA VI Reference In"=w1730, "error in"=w1729, "TTrig?"=w1731) -> ()  [unwired: 2 out]
        n1414 = local write "Initializing"(FALSE ("Initializing")) -> ()
        n1415 = local write "Triggered"(FALSE ("Triggered")) -> ()
        n1416 = local write "Waiting"(FALSE ("Waiting")) -> ()
      }
    }
    n1417 = Not(x=w1406) -> (.not. x?=w1419:bool)
    n1418 = And(x="Trap Trig. Fl.", y=w1419) -> (x .and. y?=w1416:bool)
    n1419 = local read "Tether"() -> (w1553:bool)
    n1420 = Or(x=w1416, y="Reinitialize") -> (x .or. y?=w1402:bool)
    n1421 = feedback #24(w1412) -> (w1417:string)
    n1422 = Select(t=w1412, s=w1416, f=w1417) -> (s? t:f=w1411:string)
    n1423 = Select(t=w1412, s="Reinitialize", f=w1411) -> (s? t:f=w1410:string)
    n1424 = feedback #25(0) -> (w1414:i32)
    n1425 = feedback #26(w1546) -> (w1545:dbl[])
    n1426 = Build Array (concatenate)(w1546, w1545) -> (w1370:dbl[])
    n1427 = case "For determining if there is a tether still" shown="True" w1553 {
      tunnel: w1552 -> [_ w1857]
      frame False {
      }
      frame True {
        n1428 = Greater?(x="Lost Tether Alarm Threshold (pN)", y=w1857) -> (0:w1855:bool)
        n1429 = case shown="True" w1855 {
          frame False {
          }
          frame True {
            w1858 = FALSE ("Value (Signaling)")
            n1430 = flat-sequence {
              frame #0 {
                # "stop only if saving"
                n1431 = local read "Saving..."() -> (w1870:bool)
                n1432 = And(x=w1870, y="TA Cancel Save?") -> (x .and. y?=w1869:bool)
                n1433 = local write "Stop Saving"(w1869) -> ()
              }
              frame #1 {
                n1434 = case shown="True" "TA Green Off?" {
                  frame False {
                  }
                  frame True {
                    w1873 = FALSE ("Fl. Triggered...")
                    n1435 = local write "Fl. Triggered..."(w1873) -> ()
                    n1436 = property on="Green Laser ON/Interlacing" class="Bool (strict)"("Val(Sgnl)"=w1873) -> ()  [unwired: 2 in, 2 out]
                  }
                }
              }
            }
            n1437 = local read "Time tether formed"() -> (w1864:timestamp)
            n1438 = Get Date/Time In Seconds() -> (seconds since 1Jan1904=w1865:timestamp)
            n1439 = Subtract(x=w1865, y=w1864) -> (x-y=w1863:dbl)
            n1440 = Number To Decimal String(number=w1863) -> (decimal integer string=w1860:string)  [unwired: 1 out]
            n1441 = local read "Messages"() -> (w1867:string)
            n1442 = call <vilib>:"Beep.vi"() -> ()  [unwired: 3 in, 9 out]
            n1443 = Concatenate Strings("Lost tether (" ("Message to add"), w1860, " s)." ("string")) -> (w1862:string)
            n1444 = local write "Tether"(FALSE ("Tether")) -> ()
            n1445 = call "Update messages.vi"("Message to add"=w1862, "Old message string"=w1867) -> ("New message string"=w1866:string)
            n1446 = local write "Messages"(w1866) -> ()
            n1447 = property on="Fl. Triggered..." class="Bool (strict)"("Val(Sgnl)"=w1858) -> ()  [unwired: 2 in, 2 out]
            n1448 = local write "Dip for Protein"(w1858) -> ()
            n1449 = property on="Trap Pos. FB ON" class="Bool (strict)"("Val(Sgnl)"=w1858) -> ()  [unwired: 2 in, 2 out]
            n1450 = property on="Trap Trig. Fl." class="Bool (strict)"("Val(Sgnl)"=w1858) -> ()  [unwired: 2 in, 2 out]
          }
        }
      }
    }
    n1451 = case "For triggering actions based on the trap position (e.g., turning the excitation laser on if trap under feedback moves so far)" shown="True" "Trap Trig. Fl." {
      tunnel: w1397 -> [_ w1746]
      tunnel: w1410 -> [_ w1745]
      tunnel: ["" ("t") w1744] -> w1418
      tunnel: w1402 -> [_ w1743]
      tunnel: [0 ("t") w1742] -> w1415
      tunnel: w1414 -> [_ w1741]
      tunnel: w1389 -> [_ w1740]
      tunnel: w1388 -> [_ w1739]
      frame False {
      }
      frame True {
        n1452 = case shown="\"Wait for trigger\"" w1745 {
          tunnel: w1746 -> [w1763 _ _ w1811]
          tunnel: [w1760 w1792 "" ("t") w1814] -> w1744
          tunnel: w1743 -> [_ _ _ w1802]
          tunnel: [w1759 w1789 0 ("t") w1803] -> w1742
          tunnel: w1741 -> [_ w1791 _ w1809]
          tunnel: w1740 -> [w1748 w1786 _ w1805]
          tunnel: w1739 -> [w1747 w1785 _ w1804]
          frame "Wait for trigger" {
            n1453 = local read "Trap Trig. (FPGA)"() -> (w1751:bool)
            n1454 = Subtract(x=w1763, y="Mean T1 Position\nto compare (nm)") -> (x-y=w1756:dbl[])
            n1455 = call <vilib>:"Std Deviation and Variance.vi"("X"=w1756) -> ("mean"=→"mean":dbl, "standard deviation"=→"standard\ndeviation":dbl)  [unwired: 1 in, 1 out]
            n1456 = Array Max & Min(array=w1756) -> (max value=→"max value":dbl, min value=→"min value":dbl)  [unwired: 2 out]
            n1457 = Greater?(x=w1756, y="Threshold (nm)") -> (0:w1766:bool[])
            n1458 = case shown="True" w1751 {
              tunnel: w1748 -> [_ w1772]
              tunnel: w1747 -> [_ w1771]
              tunnel: [FALSE ("TTrig?") w1770] -> w1754
              frame False {
              }
              frame True {
                n1459 = xnode "Read/Write Control"("FPGA VI Reference In"=w1772, "error in"=w1771) -> ("TTrig?"=w1770:bool)  [unwired: 2 out]
              }
            }
            n1460 = Or Array Elements(Boolean array=w1766) -> (logical OR=w1753:bool)
            n1461 = Select(t=w1754, s=w1751, f=w1753) -> (s? t:f=w1752:bool)
            n1462 = Not(x=w1751) -> (.not. x?=w1750:bool)
            n1463 = And(x=w1752, y=w1750) -> (x .and. y?=w1749:bool)
            n1464 = Select(t="Triggered", s=w1752, f="Wait for trigger") -> (s? t:f=w1760:string)
            n1465 = case shown="True" w1752 {
              tunnel: [0 0] -> w1759
              tunnel: w1748 -> [_ w1777]
              tunnel: w1747 -> [_ w1776]
              frame False {
                "Waiting" <- TRUE ("Waiting")
              }
              frame True {
                n1466 = xnode "Read/Write Control"("FPGA VI Reference In"=w1777, "error in"=w1776, "TTrig?"=FALSE) -> ()  [unwired: 2 out]
                n1467 = local read "Messages"() -> (w1780:string)
                n1468 = call <vilib>:"Beep.vi"() -> ()  [unwired: 12 in]
                n1469 = call "Update messages.vi"("Message to add"="Unwinding trigger.", "Old message string"=w1780) -> ("New message string"=w1781:string)
                n1470 = local write "Messages"(w1781) -> ()
                n1471 = local write "Waiting"(FALSE ("Waiting")) -> ()
                "Triggered" <- TRUE ("Triggered")
              }
            }
            n1472 = case "Only need to turn on laser if host triggered" shown="True" w1749 {
              frame False {
              }
              frame True {
                n1473 = property on="Green Laser ON/Interlacing" class="Bool (strict)"("Val(Sgnl)"=TRUE ("Value (Signaling)")) -> ()  [unwired: 2 in, 2 out]
              }
            }
          }
          frame "Triggered" {
            n1474 = local read "Trap Trig. (FPGA)"() -> (w1788:bool)
            n1475 = Increment(x=w1791) -> (x+1=w1789:i32)
            n1476 = Greater Or Equal?(x=w1789, y="Fl. ON time (n)") -> (x >= y?=w1787:bool)
            n1477 = Select(t="Wait for trigger", s=w1787, f="Triggered" ("t")) -> (s? t:f=w1792:string)
            n1478 = And(x=w1787, y=w1788) -> (x .and. y?=w1784:bool)
            n1479 = case shown="True" w1784 {
              tunnel: w1786 -> [_ w1796]
              tunnel: w1785 -> [_ w1795]
              frame False {
              }
              frame True {
                n1480 = xnode "Read/Write Control"("FPGA VI Reference In"=w1796, "error in"=w1795, "FPGA Trap Trig"=TRUE) -> ()  [unwired: 2 out]
              }
            }
            n1481 = case shown="True" w1787 {
              frame False {
              }
              frame True {
                w1798 = FALSE ("Value (Signaling)")
                n1482 = local write "Triggered"(w1798) -> ()
                n1483 = local write "Waiting"(TRUE ("Waiting")) -> ()
                n1484 = property on="Green Laser ON/Interlacing" class="Bool (strict)"("Val(Sgnl)"=w1798) -> ()  [unwired: 2 in, 2 out]
              }
            }
          }
          frame "Do nothing" {
          }
          frame "Initialize", Default {
            n1485 = Increment(x=w1809) -> (x+1=w1813:i32)
            n1486 = Select(t=1, s=w1802, f=w1813) -> (s? t:f=w1803:i32)
            n1487 = feedback #27(w1811) -> (w1817:dbl[])
            n1488 = Build Array (concatenate)(w1811, w1817) -> (w1810:dbl[])
            n1489 = Greater Or Equal?(x=w1803, y="Wait to get offset (n)") -> (x >= y?=w1806:bool)
            n1490 = Select(t=w1811, s=w1802, f=w1810) -> (s? t:f=w1812:dbl[])
            n1491 = feedback-in #27(w1812) -> ()
            n1492 = call-poly <vilib>:"Mean.vi"("X"=w1812) -> ("mean"=w1807:dbl)  [unwired: 1 out]
            n1493 = local write "Mean T1 Position\nto compare (nm)"(w1807) -> ()
            n1494 = case shown="True" w1802 {
              tunnel: w1805 -> [_ w1823]
              tunnel: w1804 -> [_ w1822]
              frame False {
              }
              frame True {
                w1819 = FALSE ("FPGA Trap Trig")
                n1495 = xnode "Read/Write Control"("FPGA VI Reference In"=w1823, "error in"=w1822, "FPGA Trap Trig"=w1819) -> ("FPGA VI Reference Out"=w1821:T19, "error out"=w1820:errorcluster)
                n1496 = xnode "Read/Write Control"("FPGA VI Reference In"=w1821, "error in"=w1820, "TTrig?"=w1819) -> ()  [unwired: 2 out]
              }
            }
            n1497 = Select(t="Wait for trigger", s=w1806, f="Initialize") -> (s? t:f=w1814:string)
            n1498 = case shown="True" w1806 {
              tunnel: w1807 -> [_ w1826]
              tunnel: w1805 -> [_ w1835]
              tunnel: w1804 -> [_ w1834]
              frame False {
                n1499 = local write "Waiting"(FALSE ("Waiting")) -> ()
                "Initializing" <- TRUE ("Initializing")
              }
              frame True {
                n1500 = local read "Threshold (nm)"() -> (w1838:dbl)
                n1501 = local read "AOM X Cal (nm/MHz)"() -> (w1837:dbl)
                n1502 = Add(x=w1826, y=w1838) -> (x+y=w1839:dbl)
                n1503 = Divide(x=w1839, y=w1837) -> (x/y=w1836:dbl)
                n1504 = call "IR AOM freq to word.vi"("Frequency In (MHz)"=w1836) -> ("Frequency Word Out (double)"=w1833:dbl)
                n1505 = local write "Initializing"(FALSE ("Initializing")) -> ()
                n1506 = local write "Waiting"(TRUE ("Waiting")) -> ()
                n1507 = To Quad Integer(1:w1833) -> (0:w1832:i64)
                n1508 = xnode "Read/Write Control"("FPGA VI Reference In"=w1835, "error in"=w1834, "FPGA TTrig Thresh"=w1832) -> ("FPGA VI Reference Out"=w1829:T19, "error out"=w1828:errorcluster)
                n1509 = xnode "Read/Write Control"("FPGA VI Reference In"=w1829, "error in"=w1828, "FPGA Trap Trig"=TRUE) -> ()  [unwired: 2 out]
              }
            }
          }
        }
      }
    }
    n1510 = feedback-in #24(w1418) -> ()
    n1511 = feedback-in #25(w1415) -> ()
    n1512 = Split 1D Array(array=w1370, index=w1432) -> (first subarray=w1542:dbl[])  [unwired: 1 out]
    n1513 = feedback-in #26(w1542) -> ()
    n1514 = call-poly <vilib>:"Mean.vi"("X"=w1542) -> ("mean"=w1541:dbl)  [unwired: 1 out]
    "Bead Mean (nm)" <- w1541
    n1515 = Subtract(x=w1542, y=w1541) -> (x-y=w1540:dbl[])
    n1516 = Square(x=w1540) -> (x^2=w1539:dbl[])
    n1517 = call-poly <vilib>:"Mean.vi"("X"=w1539) -> ("mean"=w1538:dbl)  [unwired: 1 out]
    n1518 = Square Root(x=w1538) -> (sqrt(x)=w1537:dbl)
    n1519 = Multiply(x=10.0, y=w1537) -> (x*y=→"RMS (Ang)":dbl)
    n1520 = xnode ("Read/Write Control")("FPGA VI Reference In"=w1575, "error in"=w1574) -> ("FPGA VI Reference Out"=w1400:T19, "error out"=w1399:errorcluster, "AI2 Y Sum Set 1"=w1673:i16, "AI2 Y Sum Set 2"=w1672:i16, "AI1 X Set 1"=w1464:fxp<+/-,16,1>, "AI1 X Set 2"=w1463:fxp<+/-,16,1>, "Trap Pos FB Int Signal"=→"Trap Pos FB Int Signal":fxp<+/-,24,9>, "Trap Pos FB Int-Norm Signal"=→"Trap Pos FB Int-Norm Signal":fxp<+/-,16,1>, "Trap Pos FB Action"=w1457:i64, "Scanning"=→"AOD Scanning":bool, "Scan I"=→"AOD Scan I":u64, "Scanning MCL"=w1675:bool, "Scan I (MCL)"=→"MCL Scan I":u64, "Green FB Sum"=w1612:i16, "Trap Pos FB Action"=w1387:i64, "TTrig Fin Thresh"=w1383:i64, "Red FB Intensity"=w1364:i16)
    "MCL Scanning" <- w1675
    "Trap Pos FB Action" <- w1457
    n1521 = local read "FB Trig Integrate"() -> (w1381:u32)
    n1522 = Divide(x=w1612, y=3276.7) -> (x/y=w1362:dbl)
    "Green laser intensity (V)" <- w1362
    n1523 = Divide(x=w1364, y=3276.7) -> (x/y=w1363:dbl)
    "Red laser intensity (V)" <- w1363
    n1524 = Divide(x=w1387, y=w1381) -> (x/y=w1380:dbl)
    "TTrig Sig (Int)" <- w1380
    n1525 = Divide(x=w1383, y=w1381) -> (x/y=w1378:dbl)
    "TTrig Fin Thresh (Int)" <- w1378
    n1526 = Bundle(w1362, w1363) -> (→"Fluorescence laser intensities plot":cluster{dbl, dbl})  [unwired: 1 in]
    n1527 = local read "AOM X Cal (nm/MHz)"() -> (w1386:dbl)
    n1528 = local read "AI2 (V)"() -> (w1674:cluster{"Set 1":dbl, "Set 2":dbl})
    n1529 = Bundle By Name(cluster=w1674, "Set 1"=w1673, "Set 2"=w1672) -> (w1670:cluster{"Set 1":dbl, "Set 2":dbl})
    n1530 = Divide(x=w1457, y=327.67) -> (x/y=→"Action (%)":dbl)
    n1531 = local read "Trap X (AI1)"() -> (w1477:T10)
    n1532 = call "IR AOM word double to freq.vi"("Frequency Word In (double)"=w1378) -> ("Frequency Out (MHz)"=w1377:dbl)
    n1533 = call "IR AOM word double to freq.vi"("Frequency Word In (double)"=w1380) -> ("Frequency Out (MHz)"=w1379:dbl)
    n1534 = Divide(x=w1670, y=3276.7) -> (x/y=w1669:cluster{"Set 1":dbl, "Set 2":dbl})
    n1535 = Multiply(x=w1379, y=w1386) -> (x*y=w1385:dbl)
    "TTrig Sig (nm)" <- w1385
    n1536 = Multiply(x=w1377, y=w1386) -> (x*y=w1384:dbl)
    "TTrig Fin Thresh (nm)" <- w1384
    n1537 = local write "AI2 (V)"(w1669) -> ()
    n1538 = Bundle(cluster=w1477, "Trap 1"=w1464, "Trap 2"=w1463) -> (→"Trap X (AI1)":T10)
    n1539 = Bundle(w1385, w1384) -> (→"TTrig":cluster{dbl, dbl})  [unwired: 1 in]
    n1540 = flat-sequence "To save data" {
      tunnel: [w2706] -> w1693
      tunnel: [w2707] -> w1692
      tunnel: w1643 -> [w2700]
      tunnel: w1405 -> [w2704]
      tunnel: ["Save Calibration"] -> w1666
      tunnel: w1663 -> [w2703]
      tunnel: [w2696] -> w1662
      tunnel: [w2693] -> w1661
      tunnel: [w2690] -> w1660
      tunnel: w1642 -> [w2692]
      tunnel: w1557 -> [w2686]
      tunnel: [w2686] -> w1556
      tunnel: ["Start Saving"] -> w1522
      tunnel: [w2680] -> w1445
      tunnel: [w2679] -> w1444
      tunnel: w1693 -> [w2942]
      tunnel: w1692 -> [w2941]
      tunnel: w1446 -> [w2940]
      tunnel: w1666 -> [w2939]
      tunnel: w1662 -> [w2937]
      tunnel: w1661 -> [w2936]
      tunnel: w1660 -> [w2935]
      tunnel: w1531 -> [w2934]
      tunnel: w1567 -> [w2933]
      tunnel: w1556 -> [w2932]
      tunnel: w1522 -> [w2931]
      tunnel: w1520 -> [w2930]
      tunnel: w1496 -> [w2929]
      tunnel: w1445 -> [w2928]
      tunnel: w1444 -> [w2927]
      tunnel: w1443 -> [w2926]
      tunnel: w1366 -> [w2925]
      frame #0 {
        n1541 = Or(x="Save N Sets", y="Start Saving") -> (x .or. y?=w2687:bool)
        n1542 = To Double Precision Float(number=w2703) -> (double precision float=w2697:dbl)
        n1543 = Build Array(w2687, "Save Calibration", w2700, w2692) -> (w2702:bool[])
        n1544 = Compound Arithmetic op=OR("Save Calibration", w2700, w2687, w2692) -> (w2705:bool)
        n1545 = Boolean Array To Number(Boolean array=w2702) -> (number=w2699:u32)
        n1546 = feedback #28(FALSE ("Save APD Data\nwith Trap Data")) -> (w2681:bool)
        n1547 = feedback #29(refnum<k0> refnum) -> (w2708:refnum<file>)
        n1548 = feedback #30(refnum<k0> refnum) -> (w2683:refnum<file>)
        n1549 = feedback #31(FALSE ("Save APD Data\nwith Trap Data")) -> (w2691:bool)
        n1550 = feedback #32(refnum<k0> refnum) -> (w2694:refnum<file>)
        n1551 = feedback #33(0) -> (w2710:i32)
        n1552 = feedback #34() -> (w2698:u32)  [unwired: 1 out]
        n1553 = case shown="True" w2705 {
          tunnel: [w2717 1] -> w2706
          tunnel: w2710 -> [w2719 _]
          tunnel: [w2718 w2737] -> w2707
          tunnel: w2708 -> [w2718 _]
          tunnel: w2704 -> [_ w2757]
          tunnel: w2697 -> [_ w2755]
          tunnel: w2699 -> [_ w2758]
          tunnel: [w2716 w2736] -> w2696
          tunnel: w2698 -> [w2716 _]
          tunnel: [w2715 w2734] -> w2693
          tunnel: w2694 -> [w2715 _]
          tunnel: [w2714 w2733] -> w2690
          tunnel: w2691 -> [w2714 _]
          tunnel: "Start Saving" -> [_ w2731]
          tunnel: w2686 -> [_ w2730]
          tunnel: [w2713 w2721] -> w2679
          tunnel: w2683 -> [w2713 _]
          tunnel: [w2712 w2720] -> w2680
          tunnel: w2681 -> [w2712 _]
          frame False {
            n1554 = Increment(x=w2719) -> (x+1=w2717:i32)
          }
          frame True {
            w2727 = FALSE ("Start Saving")
            w2732 = 9.0  # File Version
            w2740 = FALSE ("prepend array or string size? (T)")
            w2738 = T36."big-endian, network order" ("byte order (0:big-endian, network order)")
            n1555 = local read "BD 1 Frequency 1 (MHz)"() -> (w2754:dbl)
            n1556 = local read "BD 2 Frequency 1 (MHz)"() -> (w2753:dbl)
            n1557 = local read "BD 1 Frequency 2 (MHz)"() -> (w2752:dbl)
            n1558 = local read "BD 2 Frequency 2 (MHz)"() -> (w2751:dbl)
            n1559 = local read "BD 1 Frequency 3 (MHz)"() -> (w2750:dbl)
            n1560 = local read "BD 2 Frequency 3 (MHz)"() -> (w2749:dbl)
            n1561 = Array Size(array=w2730) -> (size(s)=w2729:i32)
            n1562 = To Double Precision Float(number=w2729) -> (double precision float=w2728:dbl)
            n1563 = local write "Save Calibration"(w2727) -> ()
